vi "CreateIntelliSense Control.vi"(11 "error in":errorcluster) -> (4 "IntelliSense Control":refnum<class "IntelliSenseStringControl.lvclass">, 15 "error out":errorcluster)   [LabVIEW 2016, in "StringIntelliSense.lvlib" / "IntelliSenseStringControl.lvclass"]
uses:
  IntelliSenseStringControl.lvclass
  Typedefs/String Monitor Details.ctl
  Suggestions IO/base/SuggestionIObase.lvclass
  IntelliSenseStringControl.lvclass/IntelliSenseStringControl.ctl
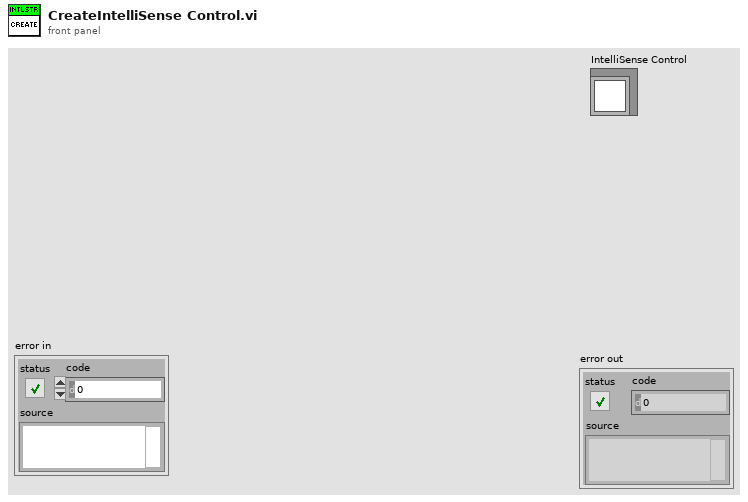
[diagram p1: front panel]
types:
  T1 = typedef "StringIntelliSense.lvlib/IntelliSenseStringControl.lvclass/String Monitor Details.ctl" = cluster{"Str Ctl Refnum":refnum<vi>, "Str ctrl Suggestion":string[], "Case Sensitive Suggestions?":bool, "Append User String to Suggestion?":bool, "Autofill Suggestion Choices?":bool, "Suggestion IO":refnum<class "SuggestionIObase.lvclass">}
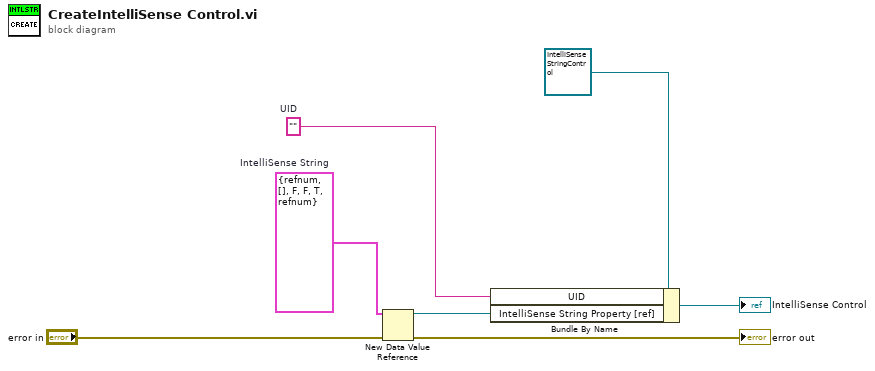
[diagram p0: block diagram]
diagram:
  w1 = ""  # UID
  w6 = T1 {"Str Ctl Refnum"=refnum, "Str ctrl Suggestion"=[], "Case Sensitive Suggestions?"=FALSE, "Append User String to Suggestion?"=FALSE, "Autofill Suggestion Choices?"=TRUE, "Suggestion IO"=refnum}  # IntelliSense String
  n1 = New Data Value Reference(data value=w6, error in="error in") -> (data value reference=w3:refnum<data-value>, error out=→"error out":errorcluster)
  n2 = Bundle By Name(cluster=refnum<class "IntelliSenseStringControl.lvclass"> refnum ("StringIntelliSense.lvlib:IntelliSense String"), "UID"=w1, "IntelliSense String Property [ref]"=w3) -> (→"IntelliSense Control":refnum<class "IntelliSenseStringControl.lvclass">)
